vi "Move Absolute (SubVI).vi"(8 "error in (no error)":errorcluster, 10 "Move to Angle":dbl, 11 "VISA Refnum in":refnum<visa-resource-name>) -> (0 "error out":errorcluster, 2 "New Angle":dbl, 3 "VISA Refnum out":refnum<visa-resource-name>)   [LabVIEW 2012]
uses:
  <instrlib>/ZaberTSeries/Public/Utility/Request.ctl
  <instrlib>/ZaberTSeries/ZaberTSeries.lvlib
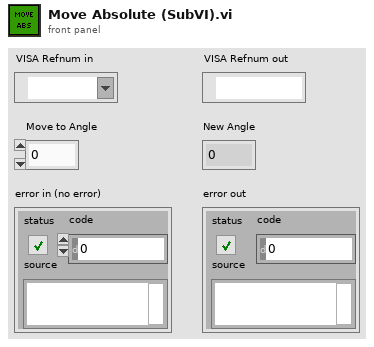
[diagram p1: front panel]
types:
  T1 = typedef "ZaberTSeries.lvlib/Request.ctl" = cluster{"Device Number":u8, "Command":u8, "Data":i32, "Response Count":i32}
  T2 = typedef "ZaberTSeries.lvlib/Response.ctl" = cluster{"Device Number":u8, "Command":u8, "Data":i32}
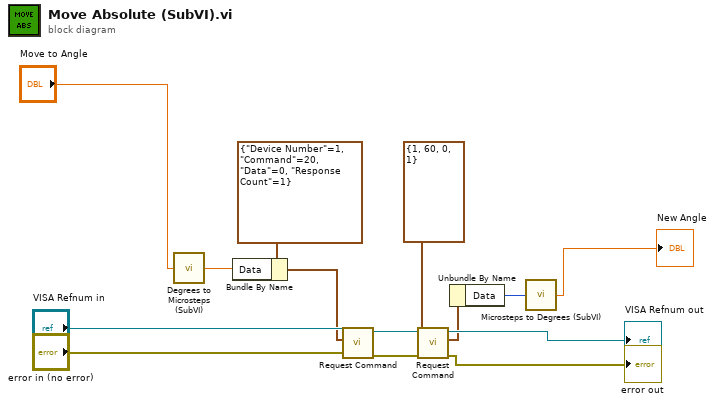
[diagram p0: block diagram]
diagram:
  n1 = call "Degrees to Microsteps (SubVI).vi"("Degrees"="Move to Angle") -> ("Microsteps"=w2:dbl)  [unwired: 4 in]
  n2 = Bundle By Name(cluster=T1 {"Device Number"=1, "Command"=20, "Data"=0, "Response Count"=1} ("Request"), "Data"=w2) -> (w3:T1)
  n3 = call <instrlib>:"Request Command.vi"("error in (no error)"="error in (no error)", "Request"=w3, "VISA resource name"="VISA Refnum in") -> ("error out"=w4:errorcluster, "VISA resource name out"=w5:refnum<visa-resource-name>)  [unwired: 5 in, 2 out]
  n4 = call <instrlib>:"Request Command.vi"("error in (no error)"=w4, "Request"=T1 {"Device Number"=1, "Command"=60, "Data"=0, "Response Count"=1}, "VISA resource name"=w5) -> ("error out"=→"error out":errorcluster, "First Response"=w7:T2, "VISA resource name out"=→"VISA Refnum out":refnum<visa-resource-name>)  [unwired: 5 in, 1 out]
  n5 = Unbundle By Name(w7) -> ("Data"=w8:i32)
  n6 = call "Microsteps to Degrees (SubVI).vi"("Microsteps"=w8) -> ("Numeric"=→"New Angle":dbl)  [unwired: 4 in]
